vi "calcCoagDose.vi"(8 "error in (no error)":errorcluster, 9 "Coagulant":T3={"flocculator volume (L)"=100.0, "clarifier volume (L)"=0.0, "dose updates per HRT"=0, "target clarified turbidity (NTU)"=0.3, "Coagulant mode"=enum."manual", "Coag dose [mg/L]"=0.0, "pump mL/rev"=0.0, "clarifier flow [L/s]"=0.5, "min Coag dose [mg/L]"=0.0, "max Coag dose [mg/L]"=0.0, "Steps"=3, "HRT response delay"=1, "Ku*"=1.0, "DOM coag demand [mg/L]"=0.0, "min DOM coag demand [mg/L]"=0.0, "max DOM coag demand [mg/L]"=0.0} {"max DOM coag demand [mg/L]" min=0.0 max=20.0 step=0.1; "min DOM coag demand [mg/L]" min=0.0 max=10.0 step=0.1; "DOM coag demand [mg/L]" min=0.0 max=20.0 step=0.1; "HRT response delay" min=1 max=10 step=1; "Steps" min=3 step=1; "clarifier flow [L/s]" min=0.0001 max=1.0 step=0.0001; "target clarified turbidity (NTU)" min=0.1 max=5.0 step=0.01; "dose updates per HRT" min=1 max=100 step=1}, 10 "averaged data":T2) -> (0 "error out":errorcluster, 5 "coag model":T1)   [LabVIEW 2019]
uses:
  Sensor buffer command.ctl
  model type.ctl
  data cluster.ctl
  coag.ctl
panel:
  # "ramp controls"
  # "min"
  # "max"
  # "min"
  # "max"
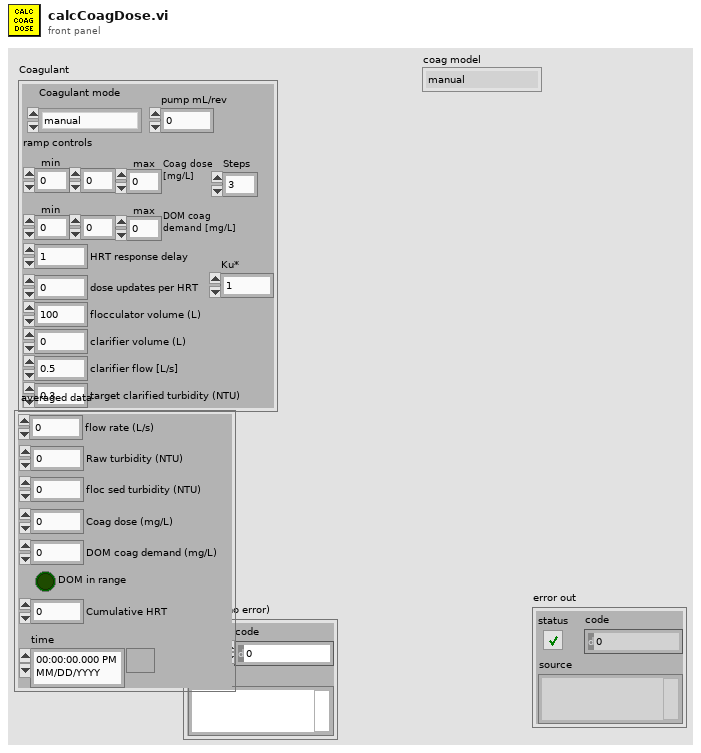
[diagram p1: front panel]
types:
  T1 = typedef "model type.ctl" = enum16{"manual", "ramp", "simple corrector"}
  T2 = typedef "data cluster.ctl" = cluster{"floc sed turbidity (NTU)":dbl, "Raw turbidity (NTU)":dbl, "flow rate (L/s)":dbl, "time":timestamp, "Cumulative HRT":dbl, "Coag dose (mg/L)":dbl, "DOM coag demand (mg/L)":dbl, "DOM in range":bool}
  T3 = typedef "coag.ctl" = cluster{"flocculator volume (L)":dbl, "clarifier volume (L)":dbl, "dose updates per HRT":u16, "target clarified turbidity (NTU)":dbl, "Coagulant mode":T1, "Coag dose [mg/L]":dbl, "pump mL/rev":dbl, "clarifier flow [L/s]":dbl, "min Coag dose [mg/L]":dbl, "max Coag dose [mg/L]":dbl, "Steps":u16, "HRT response delay":u32, "Ku*":dbl, "DOM coag demand [mg/L]":dbl, "min DOM coag demand [mg/L]":dbl, "max DOM coag demand [mg/L]":dbl}
  T4 = typedef "Sensor buffer command.ctl" = enum16{"set buffer size", "write", "refill buffer", "read recent", "read all", "read at delta HRT", "clear"}
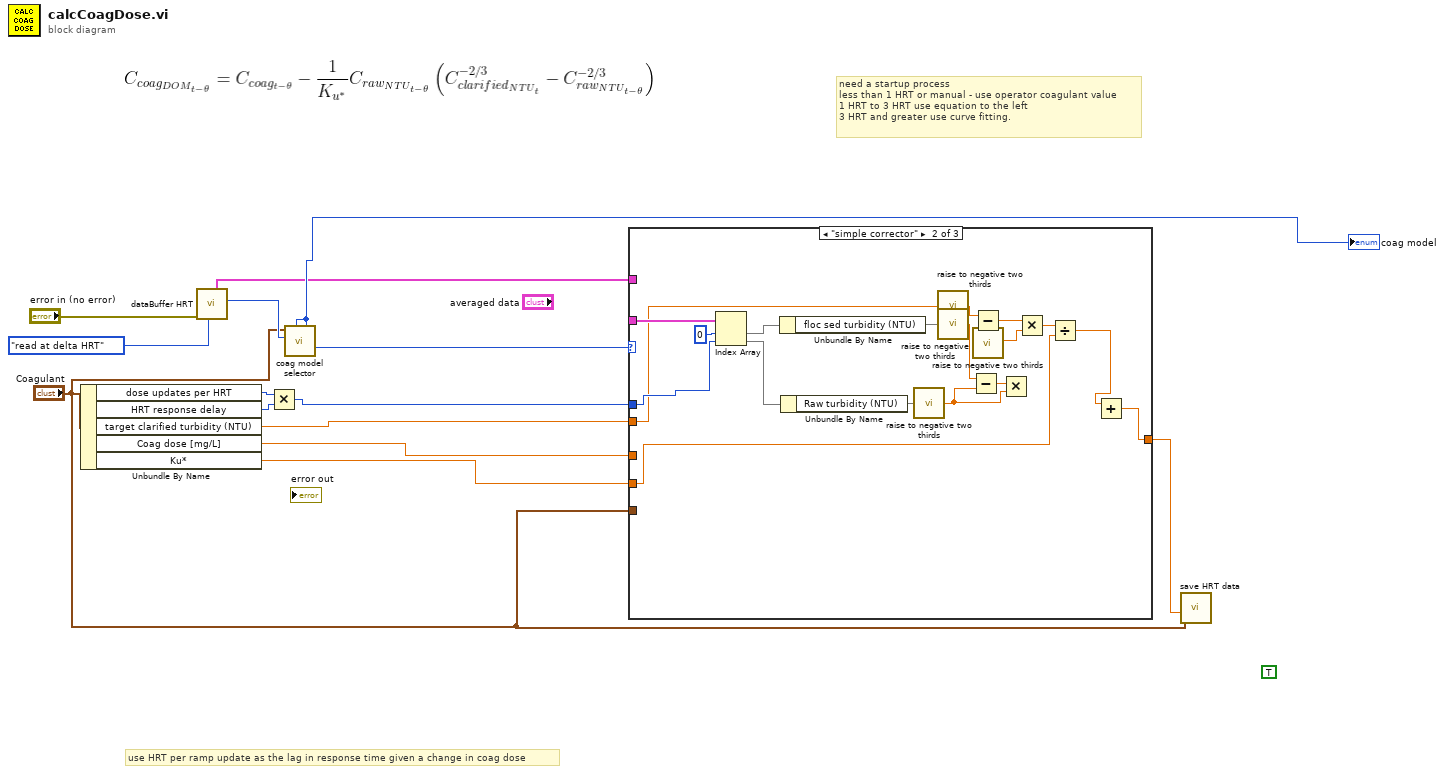
[diagram p0: block diagram]
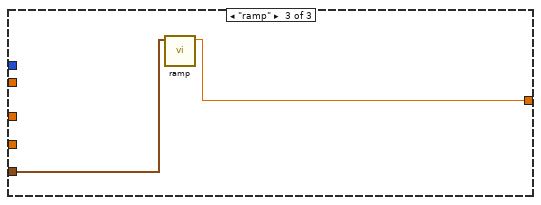
[diagram p3: hidden frame]
diagram:
  (unwired) TRUE
  # "use HRT per ramp update as the lag in response time given a change in coag dose"
  # "need a startup process \nless than 1 HRT or manual - use operator coagulant value\n1 HRT to 3 HRT use equation to the left\n3 HRT and greater use curve fitting."
  n1 = Unbundle By Name("Coagulant") -> ("dose updates per HRT"=w5:u16, "HRT response delay"=w4:u32, "target clarified turbidity (NTU)"=w9:dbl, "Coag dose [mg/L]"=w10:dbl, "Ku*"=w2:dbl)
  n2 = call "dataBuffer HRT.vi"("command"=Sensor_buffer_command."read at delta HRT", "error in (no error)"="error in (no error)") -> ("scans"=w8:i32, "recent at deltaHRT"=w1:T2)  [unwired: 5 in, 3 out]
  n3 = Multiply(x=w5, y=w4) -> (x*y=w3:u32)
  n4 = call "coag model selector.vi"("scans"=w8, "Coagulant"="Coagulant") -> ("coag model"=w13:T1)  [unwired: 9 in]
  "coag model" <- w13
  n5 = case shown="\"simple corrector\"" w13 {
    tunnel: _ -> [_ w32 _]
    tunnel: w3 -> [_ w28 _]
    tunnel: w9 -> [_ w25 _]
    tunnel: [w14 w16 w33] -> w6
    tunnel: w10 -> [w14 _ _]
    tunnel: "Coagulant" -> [_ _ w34]
    tunnel: w2 -> [_ w18 _]
    tunnel: w1 -> [_ _ _]
    frame "manual", Default {
    }
    frame "simple corrector" {
      n6 = Index Array(array=w32, index #1=0 ("index"), index #2=w28) -> (element #1=w30, element #2=w29)
      n7 = Unbundle By Name(w30) -> ("floc sed turbidity (NTU)"=w27)
      n8 = Unbundle By Name(w29) -> ("Raw turbidity (NTU)"=w26)
      n9 = call "raise to negative two thirds.vi"("Numeric in"=w26) -> ("Numeric out"=w19:dbl)  [unwired: 4 in]
      n10 = call "raise to negative two thirds.vi"("Numeric in"=w25) -> ("Numeric out"=w24:dbl)  [unwired: 4 in]
      n11 = call "raise to negative two thirds.vi"("Numeric in"=w27) -> ("Numeric out"=w23:dbl)  [unwired: 4 in]
      n12 = Subtract(x=w23, y=w19) -> (x-y=w20:dbl)
      n13 = call "raise to negative two thirds.vi"() -> ("Numeric out"=w21:dbl)  [unwired: 5 in]
      n14 = Subtract(x=w24, y=w21) -> (x-y=w22:dbl)
      n15 = Multiply(x=w20, y=w19) -> ()  [unwired: 1 out]
      n16 = Multiply(x=w22, y=w21) -> (x*y=w15:dbl)
      n17 = Divide(x=w15, y=w18) -> (x/y=w17:dbl)
      n18 = Add(x=w17) -> (x+y=w16:dbl)  [unwired: 1 in]
    }
    frame "ramp" {
      n19 = call "ramp.vi"("Coagulant"=w34) -> ("Coag dose"=w33:dbl)  [unwired: 10 in]
    }
  }
  n20 = call "save HRT data.vi"("coagulant dose"=w6, "Coagulant"="Coagulant") -> ()  [unwired: 10 in]
